vi "Show_STS_Error.vi"(8 "error in (no error)":errorcluster, 10 "Error":i32) -> (0 "error out":errorcluster)   [LabVIEW 2017]
doc: "Show error code for STS"
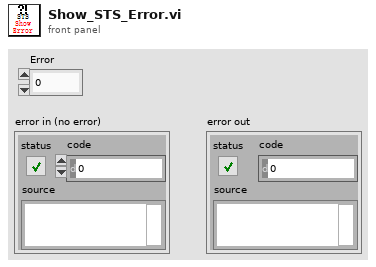
[diagram p1: front panel]
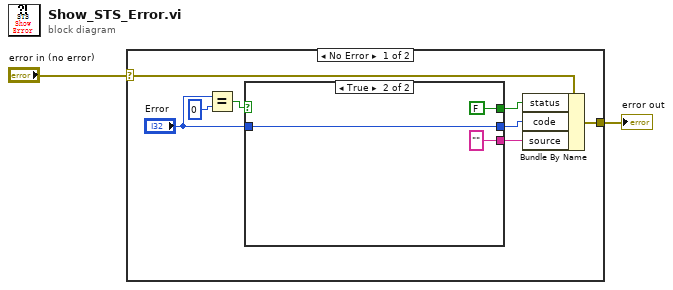
[diagram p0: block diagram]
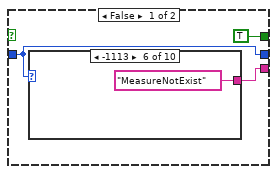
[diagram p2: hidden frame]
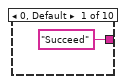
[diagram p3: hidden frame]
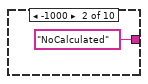
[diagram p4: hidden frame]
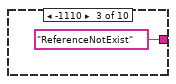
[diagram p5: hidden frame]
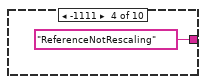
[diagram p6: hidden frame]
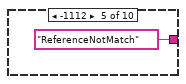
[diagram p7: hidden frame]
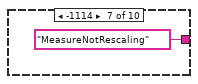
[diagram p8: hidden frame]
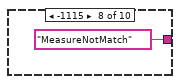
[diagram p9: hidden frame]
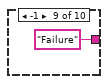
[diagram p10: hidden frame]
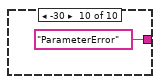
[diagram p11: hidden frame]
diagram:
  n1 = case shown="No Error" "error in (no error)" {
    selector: "error in (no error)" -> [w7 w27]
    tunnel: [w5 w27] -> w1
    frame No Error {
      n2 = Equal?(x="Error", y=0) -> (x = y?=w10:bool)
      n3 = case shown="True" w10 {
        tunnel: "Error" -> [w12 w25]
        tunnel: [w13 ""] -> w8
        tunnel: [w12 w25] -> w6
        tunnel: [TRUE FALSE] -> w3
        frame False {
          n4 = case shown="-1113" w12 {
            tunnel: ["Succeed" "NoCalculated" "ReferenceNotExist" "ReferenceNotRescaling" "ReferenceNotMatch" "MeasureNotExist" "MeasureNotRescaling" "MeasureNotMatch" "Failure" "ParameterError"] -> w13
            frame 0, Default {
            }
            frame -1000 {
            }
            frame -1110 {
            }
            frame -1111 {
            }
            frame -1112 {
            }
            frame -1113 {
            }
            frame -1114 {
            }
            frame -1115 {
            }
            frame -1 {
            }
            frame -30 {
            }
          }
        }
        frame True {
        }
      }
      n5 = Bundle By Name(cluster=w7, "status"=w3, "code"=w6, "source"=w8) -> (w5:errorcluster)
    }
    frame Error {
    }
  }
  "error out" <- w1
